vi "scaling_coeffs_tofile.vi"(10 "channel number":i32, 11 "appended path":path) -> (0 "error out":errorcluster)   [LabVIEW 2015]
panel:
  in  "Cluster":T1
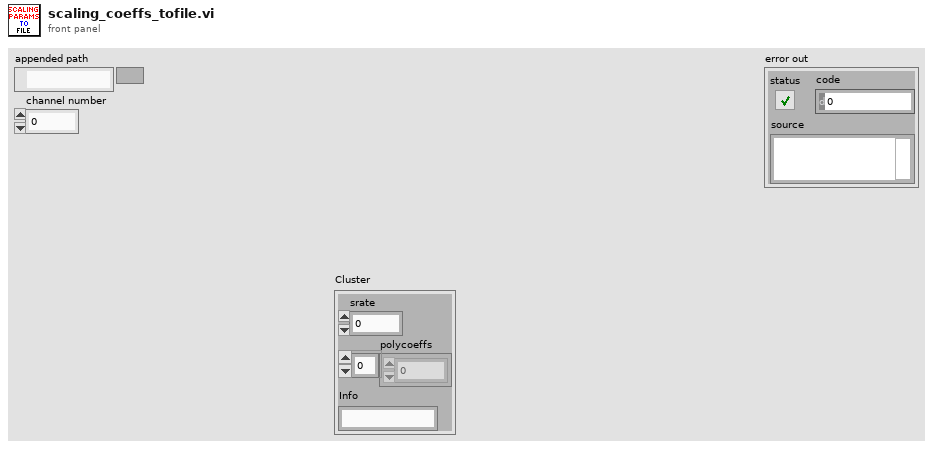
[diagram p1: front panel]
types:
  T1 = cluster{"srate":dbl, "polycoeffs":dbl[], "Info":string}
  T2 = cluster{" AI":refnum<k21>, "E_AI":errorcluster, "header":dbl[]}
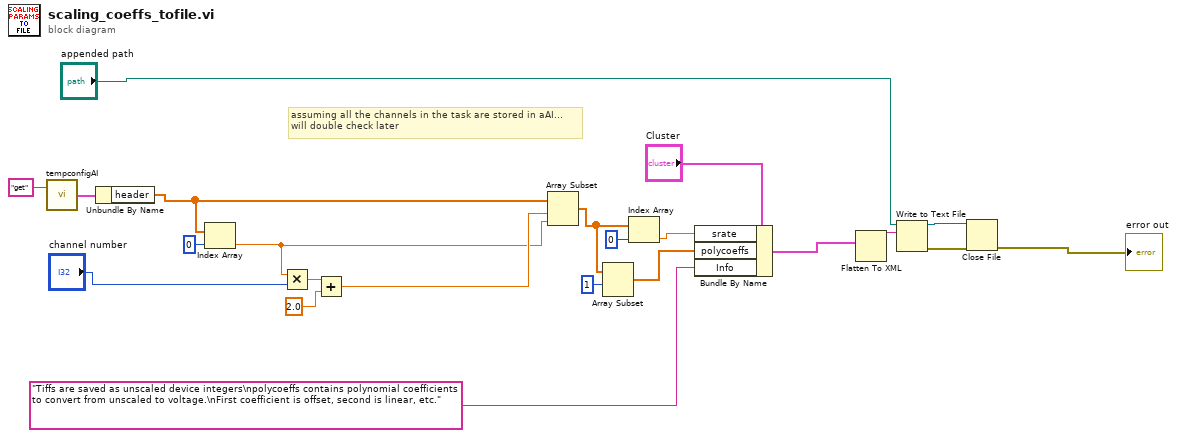
[diagram p0: block diagram]
diagram:
  # "assuming all the channels in the task are stored in aAI...\nwill double check later"
  n1 = call "tempconfigAI.vi"("command"="get") -> ("Temp Config out"=w21:T2)  [unwired: 1 in]
  n2 = Unbundle By Name(w21) -> ("header"=w17:dbl[])
  n3 = Index Array(array=w17, index=0) -> (element=w1:dbl)
  n4 = Multiply(x=w1, y="channel number") -> (x*y=w14:dbl)
  n5 = Add(x=w14, y=2.0) -> (x+y=w12:dbl)
  n6 = Array Subset(array=w17, index=w12, length=w1) -> (w6:dbl[])
  n7 = Array Subset(array=w6, index=1) -> (w7:dbl[])  [unwired: 1 in]
  n8 = Index Array(array=w6, index=0) -> (element=w8:dbl)
  n9 = Bundle By Name(cluster="Cluster", "srate"=w8, "polycoeffs"=w7, "Info"="Tiffs are saved as unscaled device integers\npolycoeffs contains polynomial coefficients to convert from unscaled to voltage.\nFirst coefficient is offset, second is linear, etc.") -> (w5:T1)
  n10 = Flatten To XML(anything=w5) -> (xml string=w20:string)
  n11 = Write to Text File(file (use dialog)="appended path", text=w20) -> (refnum out=w19:refnum<file>, error out=w18:errorcluster)  [unwired: 2 in, 1 out]
  n12 = Close File(refnum=w19, error in=w18) -> (error out=→"error out":errorcluster)  [unwired: 1 out]
